vi "AVTCP-Read Settings.vi"() -> (4 "TCP":cluster{"IP Address":string, "Port":i32}, 15 "error out":errorcluster)   [LabVIEW 2020]
uses:
  <vilib>/Utility/config.llb/Read Key (String).vi
  <vilib>/Utility/config.llb/Read Key (I32).vi
  <vilib>/Utility/config.llb/NI_LVConfig.lvlib
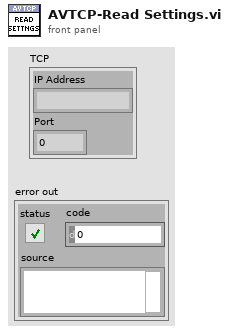
[diagram p1: front panel]
types:
  T1 = typedef "NI_LVConfig.lvlib/Config Data RefNum.ctl" = refnum<k1>
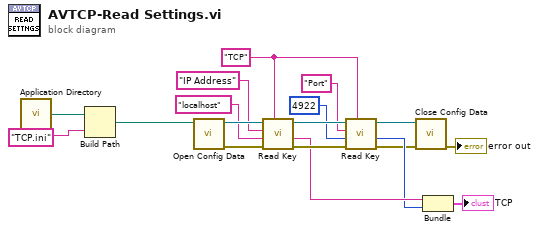
[diagram p0: block diagram]
diagram:
  w9 = "TCP" ("section")
  n1 = call <vilib>:"Application Directory.vi"() -> ("Application Directory"=w18:path)
  n2 = Build Path(base path=w18, name or relative path="TCP.ini") -> (appended path=w16:path)
  n3 = call <vilib>:"Open Config Data.vi"("configuration file path"=w16) -> ("error out"=w14:errorcluster, "refnum"=w15:T1)  [unwired: 8 in, 1 out]
  n4 = call-poly <vilib>:"Read Key.vi"("section"=w9, "error in (no error)"=w14, "default value"="localhost", "key"="IP Address", "refnum"=w15) -> ("error out"=w10:errorcluster, "value"=w6:string, "refnum out"=w11:T1)  [unwired: 3 in, 1 out]
  n5 = call-poly <vilib>:"Read Key.vi"("section"=w9, "error in (no error)"=w10, "default value"=4922, "key"="Port", "refnum"=w11) -> ("error out"=w3:errorcluster, "value"=w5:i32, "refnum out"=w2:T1)  [unwired: 3 in, 1 out]
  n6 = call <vilib>:"Close Config Data.vi"("error in (no error)"=w3, "refnum"=w2) -> ("error out"=→"error out":errorcluster)  [unwired: 8 in, 1 out]
  n7 = Bundle("value"=w6, "value"=w5) -> (→"TCP":cluster{"value":string, "value":i32})  [unwired: 1 in]
